vi "ReportPart.vi"(6 "试验项目":enum32{"静态标定", "动态优化", "程序复检", "程序固化"}(ring), 8 "error in":errorcluster, 9 "索引":i32=3, 10 "合格":T1, 11 "report in":refnum<class "NI_report.lvclass">) -> (0 "error out 2":errorcluster caption="error out", 1 "索引OUT":i32, 3 "report out":refnum<class "NI_report.lvclass">)   [LabVIEW 2020]
uses:
  <vilib>/Utility/NIReport.llb/NI_report.lvclass
  OK.ctl
  <vilib>/Utility/NIReport.llb/image depth.ctl
  <vilib>/addons/_office/_exclsub.llb/font.ctl
  Global_Variable/Global.vi
  <vilib>/Utility/NIReport.llb/Append Report Text (str wrap).vi
  <vilib>/addons/_office/word.llb/Word Easy Table (str).vi
  Global_Variable/A180648.vi
  <vilib>/Utility/NIReport.llb/NI_ReportGenerationCore.lvlib
  <vilib>/addons/_office/NI_ReportGenerationToolkit.lvlib
  <vilib>/Utility/NIReport.llb/Word/NI_Word.lvclass
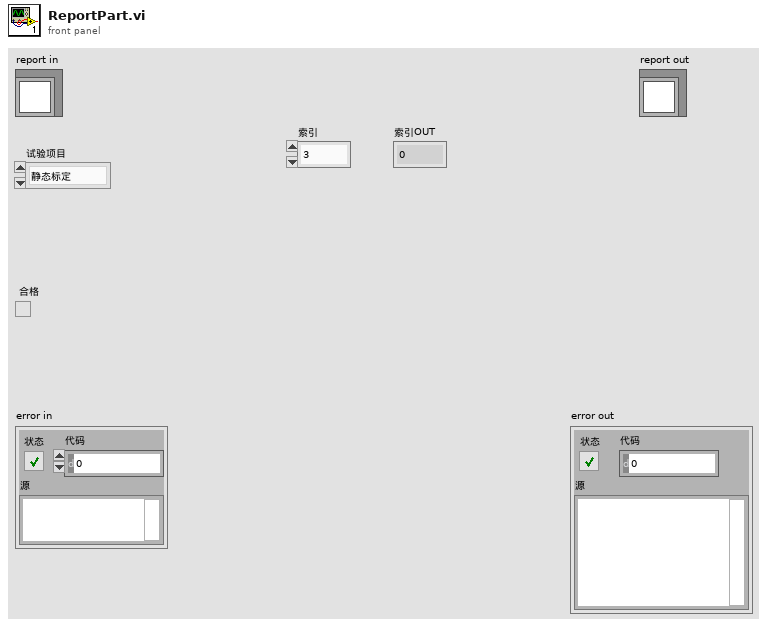
[diagram p1: front panel]
types:
  T1 = typedef "OK.ctl" = bool
  T2 = cluster{"Charset (-1)":i16, "Weight (-1)":i16, "Name":string, "Size":string}
  T3 = cluster{"Italic":enum16{"Italic Unchanged", "Italic On", "Italic Off"}, "Strike Through":enum16{"Strike Through Unchanged", "Strike Through On", "Strike Through Off"}, "Underline":enum16{"Underline Unchanged", "Underline On", "Underline Off"}, "Bold":enum16{"Bold Unchanged", "Bold On", "Bold Off"}}
  T4 = typedef "NI_ReportGenerationToolkit.lvlib/font.ctl" = cluster{"font name":string, "font size":dbl, "bold":u16, "italic":u16, "underline":u16, "strike through":u16, "font color":u32}
  T5 = typedef "NI_ReportGenerationCore.lvlib/image depth.ctl" = u16
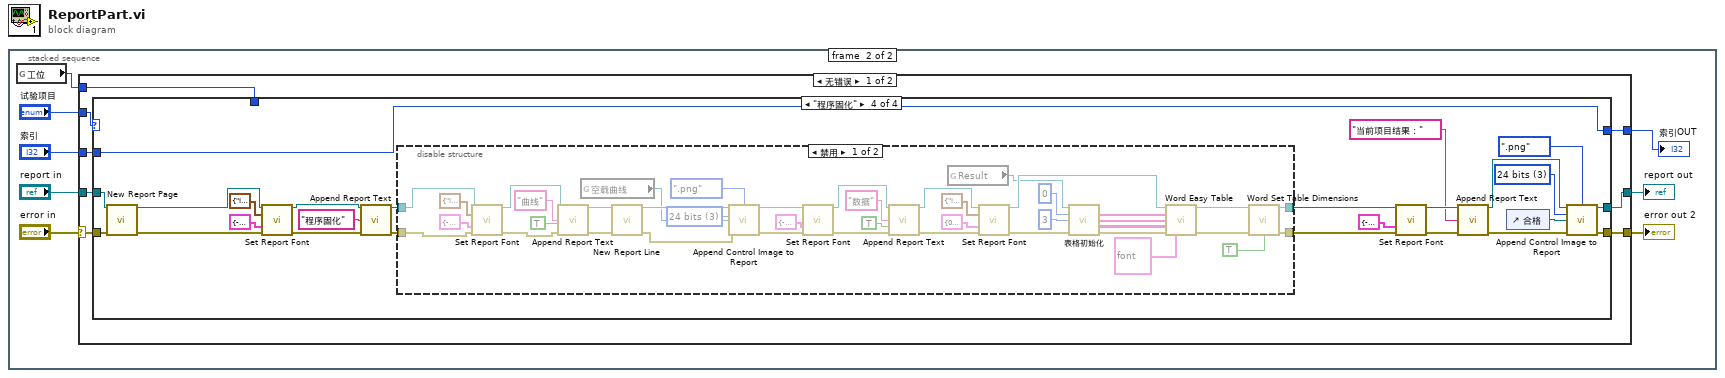
[diagram p0: block diagram]
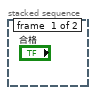
[diagram p2: hidden frame]
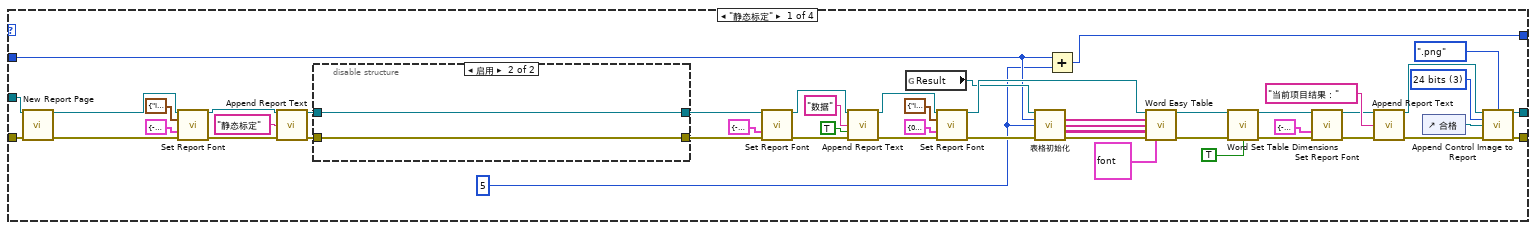
[diagram p3: hidden frame]
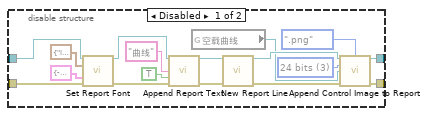
[diagram p4: hidden frame]
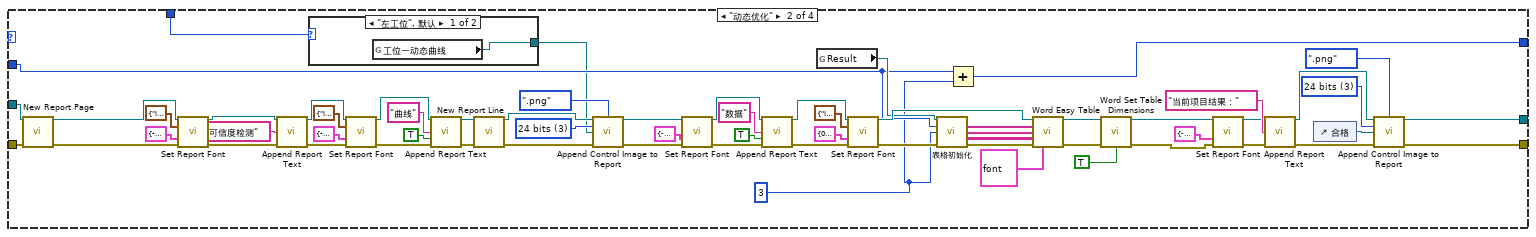
[diagram p5: hidden frame]
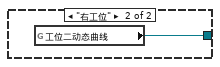
[diagram p6: hidden frame]
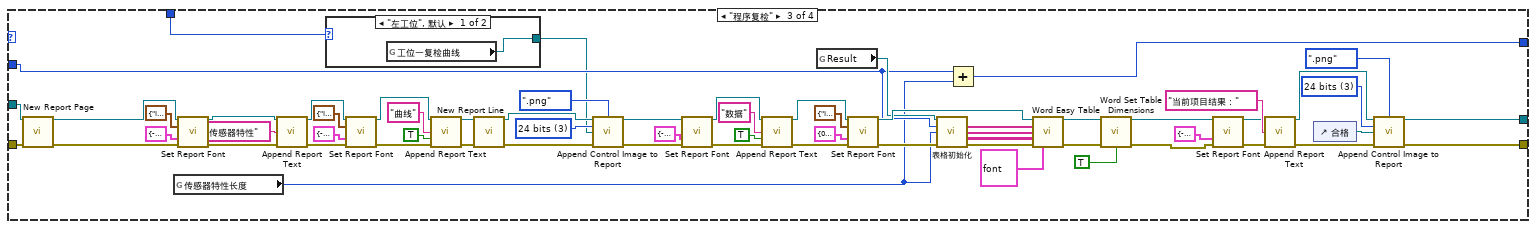
[diagram p7: hidden frame]
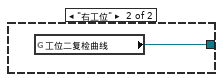
[diagram p8: hidden frame]
diagram:
  n1 = stacked-sequence {
    frame #0 {
    }
    frame #1 {
      n2 = global read "Global.vi" "工位"() -> (w1:enum16{"左工位", "右工位"})
      n3 = case shown="无错误" "error in" {
        selector: "error in" -> [w16 w285]
        tunnel: [w15 w285] -> w7
        tunnel: "试验项目" -> [w12 _]
        tunnel: [w14 w284] -> w5
        tunnel: "report in" -> [w13 w284]
        tunnel: "索引" -> [w11 w283]
        tunnel: [w10 w283] -> w2
        tunnel: w1 -> [w9 _]
        frame No Error {
          n4 = case shown="\"程序固化\"" w12 {
            tunnel: w16 -> [w59 w141 w206 w233]
            tunnel: [w54 w136 w201 w228] -> w15
            tunnel: [w23 w93 w158 w220] -> w14
            tunnel: w13 -> [w22 w92 w157 w219]
            tunnel: w11 -> [w19 w89 w154 w215]
            tunnel: [w18 w88 w153 w215] -> w10
            tunnel: w9 -> [_ w87 w152 _]
            frame "静态标定" {
              w17 = 5
              w52 = T5 3 items=["B&W", "4 bits", "8 bits", "24 bits"] ("image depth")
              n5 = call-dynamic "New Report Page.vi"("report in"=w22, "error in (no error)"=w59) -> ("report out"=w57:refnum<class "NI_report.lvclass">, "error out"=w58:errorcluster)  [unwired: 12 in]
              n6 = call-dynamic "Set Report Font.vi"("report in"=w57, "text options"=T3 {"Italic"=enum."Italic Unchanged", "Strike Through"=enum."Strike Through Unchanged", "Underline"=enum."Underline Unchanged", "Bold"=enum."Bold On"}, "font settings"=T2 {"Charset (-1)"=-1, "Weight (-1)"=-1, "Name"="楷体", "Size"="16 "}, "error in (no error)"=w58) -> ("report out"=w65:refnum<class "NI_report.lvclass">, "error out"=w64:errorcluster)  [unwired: 9 in, 1 out]
              n7 = call-poly <vilib>:"Append Report Text.vi"("report in"=w65, "text"="静态标定", "error in (no error)"=w64) -> ("report out"=w61:refnum<class "NI_report.lvclass">, "error out"=w60:errorcluster)  [unwired: 9 in, 2 out]
              n8 = disable-structure shown="启用" {
                disable-tunnel: w61 -> [w82 w84]
                disable-tunnel: w60 -> [w81 w83]
                disable-tunnel: [w77 w84] -> w41
                disable-tunnel: [w76 w83] -> w39
                frame Disabled {
                  w78 = T5 3 items=["B&W", "4 bits", "8 bits", "24 bits"] ("image depth")
                  n9 = call-dynamic "Set Report Font.vi"("report in"=w82, "text options"=T3 {"Italic"=enum."Italic Unchanged", "Strike Through"=enum."Strike Through Unchanged", "Underline"=enum."Underline Unchanged", "Bold"=enum."Bold Off"}, "font settings"=T2 {"Charset (-1)"=-1, "Weight (-1)"=-1, "Name"="宋体", "Size"="12 "}, "error in (no error)"=w81) -> ("report out"=w73:refnum<class "NI_report.lvclass">, "error out"=w70:errorcluster)  [unwired: 9 in, 1 out]
                  n10 = call-poly <vilib>:"Append Report Text.vi"("report in"=w73, "text"="曲线", "append on new line? (F)"=TRUE, "error in (no error)"=w70) -> ("report out"=w72:refnum<class "NI_report.lvclass">, "error out"=w71:errorcluster)  [unwired: 8 in, 2 out]
                  n11 = global read "A180648.vi" "空载曲线"() -> (w66:refnum<vi>)
                  n12 = call-dynamic "New Report Line.vi"("report in"=w72, "error in (no error)"=w71) -> ("report out"=w79:refnum<class "NI_report.lvclass">, "error out"=w80:errorcluster)  [unwired: 12 in]
                  n13 = call-dynamic "Append Control Image to Report.vi"("report in"=w79, "image file type (.jpg)"=enum16{".jpg", ".png"}.".png", "image depth"=w78, "ctrl reference"=w66, "error in (no error)"=w80) -> ("report out"=w77:refnum<class "NI_report.lvclass">, "error out"=w76:errorcluster)  [unwired: 7 in, 2 out]
                }
                frame Enabled {
                }
              }
              n14 = call-dynamic "Set Report Font.vi"("report in"=w41, "font settings"=T2 {"Charset (-1)"=-1, "Weight (-1)"=-1, "Name"="宋体", "Size"="12 "}, "error in (no error)"=w39) -> ("report out"=w42:refnum<class "NI_report.lvclass">, "error out"=w40:errorcluster)  [unwired: 10 in, 1 out]
              n15 = call-poly <vilib>:"Append Report Text.vi"("report in"=w42, "text"="数据", "append on new line? (F)"=TRUE, "error in (no error)"=w40) -> ("report out"=w26:refnum<class "NI_report.lvclass">, "error out"=w25:errorcluster)  [unwired: 8 in, 2 out]
              n16 = global read "Global.vi" "Result"() -> (w24:refnum<vi>)
              n17 = call-dynamic "Set Report Font.vi"("report in"=w26, "text options"=T3 {"Italic"=enum."Italic Unchanged", "Strike Through"=enum."Strike Through Unchanged", "Underline"=enum."Underline Unchanged", "Bold"=enum."Bold Unchanged"}, "font settings"=T2 {"Charset (-1)"=0, "Weight (-1)"=-1, "Name"="微软雅黑", "Size"="12 "}, "error in (no error)"=w25) -> ("report out"=w28:refnum<class "NI_report.lvclass">, "error out"=w27:errorcluster)  [unwired: 9 in, 1 out]
              n18 = call "表格初始化.vi"("表格引用"=w24, "索引"=w19, "长度"=w17, "错误输入（无错误）"=w27) -> ("行首字符串[]"=w30:string[], "列首字符串[]"=w29:string[], "文本数据"=w32:string[][], "错误输出"=w35:errorcluster)  [unwired: 7 in, 1 out]
              n19 = Add(x=w19, y=w17) -> (x+y=w18:i32)
              n20 = call-poly <vilib>:"Word Easy Table.vi"("report in"=w28, "row headers"=w30, "column headers"=w29, "data"=w32, "error in (no error)"=w35, "font"=T4 {"font name"="宋体", "font size"=12.0, "bold"=2, "italic"=2, "underline"=2, "strike through"=2, "font color"=16777216}) -> ("report out"=w33:refnum<class "NI_report.lvclass">, "error out"=w34:errorcluster)  [unwired: 7 in, 1 out]
              n21 = call <vilib>:"Word Set Table Dimensions.vi"("report in"=w33, "error in (no error)"=w34, "fit to page width? (F)"=TRUE) -> ("report out"=w47:refnum<class "NI_report.lvclass">, "error out"=w46:errorcluster)  [unwired: 11 in]
              n22 = call-dynamic "Set Report Font.vi"("report in"=w47, "font settings"=T2 {"Charset (-1)"=-1, "Weight (-1)"=-1, "Name"="宋体", "Size"="16 "}, "error in (no error)"=w46) -> ("report out"=w50:refnum<class "NI_report.lvclass">, "error out"=w51:errorcluster)  [unwired: 10 in, 1 out]
              n23 = call-poly <vilib>:"Append Report Text.vi"("report in"=w50, "text"="当前项目结果：", "error in (no error)"=w51) -> ("report out"=w56:refnum<class "NI_report.lvclass">, "error out"=w55:errorcluster)  [unwired: 9 in, 2 out]
              n24 = control-ref of="合格"() -> (w21:refnum<vi>)
              n25 = call-dynamic "Append Control Image to Report.vi"("report in"=w56, "image file type (.jpg)"=enum16{".jpg", ".png"}.".png", "image depth"=w52, "ctrl reference"=w21, "error in (no error)"=w55) -> ("report out"=w23:refnum<class "NI_report.lvclass">, "error out"=w54:errorcluster)  [unwired: 7 in, 2 out]
            }
            frame "动态优化" {
              w85 = 3
              w125 = T5 3 items=["B&W", "4 bits", "8 bits", "24 bits"] ("image depth")
              w134 = T5 3 items=["B&W", "4 bits", "8 bits", "24 bits"] ("image depth")
              n26 = call-dynamic "New Report Page.vi"("report in"=w92, "error in (no error)"=w141) -> ("report out"=w139:refnum<class "NI_report.lvclass">, "error out"=w140:errorcluster)  [unwired: 12 in]
              n27 = call-dynamic "Set Report Font.vi"("report in"=w139, "text options"=T3 {"Italic"=enum."Italic Unchanged", "Strike Through"=enum."Strike Through Unchanged", "Underline"=enum."Underline Unchanged", "Bold"=enum."Bold On"}, "font settings"=T2 {"Charset (-1)"=-1, "Weight (-1)"=-1, "Name"="楷体", "Size"="16 "}, "error in (no error)"=w140) -> ("report out"=w147:refnum<class "NI_report.lvclass">, "error out"=w146:errorcluster)  [unwired: 9 in, 1 out]
              n28 = call-poly <vilib>:"Append Report Text.vi"("report in"=w147, "text"="可信度检测", "error in (no error)"=w146) -> ("report out"=w143:refnum<class "NI_report.lvclass">, "error out"=w142:errorcluster)  [unwired: 9 in, 2 out]
              n29 = case shown="\"左工位\", 默认" w87 {
                tunnel: [w148 w149] -> w86
                frame "左工位", Default {
                  n30 = global read "A180648.vi" "工位一动态曲线"() -> (w148:refnum<vi>)
                }
                frame "右工位" {
                  n31 = global read "A180648.vi" "工位二动态曲线"() -> (w149:refnum<vi>)
                }
              }
              n32 = call-dynamic "Set Report Font.vi"("report in"=w143, "text options"=T3 {"Italic"=enum."Italic Unchanged", "Strike Through"=enum."Strike Through Unchanged", "Underline"=enum."Underline Unchanged", "Bold"=enum."Bold Off"}, "font settings"=T2 {"Charset (-1)"=-1, "Weight (-1)"=-1, "Name"="宋体", "Size"="12 "}, "error in (no error)"=w142) -> ("report out"=w112:refnum<class "NI_report.lvclass">, "error out"=w109:errorcluster)  [unwired: 9 in, 1 out]
              n33 = call-poly <vilib>:"Append Report Text.vi"("report in"=w112, "text"="曲线", "append on new line? (F)"=TRUE, "error in (no error)"=w109) -> ("report out"=w111:refnum<class "NI_report.lvclass">, "error out"=w110:errorcluster)  [unwired: 8 in, 2 out]
              n34 = call-dynamic "New Report Line.vi"("report in"=w111, "error in (no error)"=w110) -> ("report out"=w126:refnum<class "NI_report.lvclass">, "error out"=w127:errorcluster)  [unwired: 12 in]
              n35 = call-dynamic "Append Control Image to Report.vi"("report in"=w126, "image file type (.jpg)"=enum16{".jpg", ".png"}.".png", "image depth"=w125, "ctrl reference"=w86, "error in (no error)"=w127) -> ("report out"=w120:refnum<class "NI_report.lvclass">, "error out"=w118:errorcluster)  [unwired: 7 in, 2 out]
              n36 = call-dynamic "Set Report Font.vi"("report in"=w120, "font settings"=T2 {"Charset (-1)"=-1, "Weight (-1)"=-1, "Name"="宋体", "Size"="12 "}, "error in (no error)"=w118) -> ("report out"=w121:refnum<class "NI_report.lvclass">, "error out"=w119:errorcluster)  [unwired: 10 in, 1 out]
              n37 = call-poly <vilib>:"Append Report Text.vi"("report in"=w121, "text"="数据", "append on new line? (F)"=TRUE, "error in (no error)"=w119) -> ("report out"=w96:refnum<class "NI_report.lvclass">, "error out"=w95:errorcluster)  [unwired: 8 in, 2 out]
              n38 = global read "Global.vi" "Result"() -> (w94:refnum<vi>)
              n39 = call-dynamic "Set Report Font.vi"("report in"=w96, "text options"=T3 {"Italic"=enum."Italic Unchanged", "Strike Through"=enum."Strike Through Unchanged", "Underline"=enum."Underline Unchanged", "Bold"=enum."Bold Unchanged"}, "font settings"=T2 {"Charset (-1)"=0, "Weight (-1)"=-1, "Name"="微软雅黑", "Size"="12 "}, "error in (no error)"=w95) -> ("report out"=w98:refnum<class "NI_report.lvclass">, "error out"=w97:errorcluster)  [unwired: 9 in, 1 out]
              n40 = call "表格初始化.vi"("表格引用"=w94, "索引"=w89, "长度"=w85, "错误输入（无错误）"=w97) -> ("行首字符串[]"=w101:string[], "列首字符串[]"=w100:string[], "文本数据"=w103:string[][], "错误输出"=w106:errorcluster)  [unwired: 7 in, 1 out]
              n41 = Add(x=w89, y=w85) -> (x+y=w88:i32)
              n42 = call-poly <vilib>:"Word Easy Table.vi"("report in"=w98, "row headers"=w101, "column headers"=w100, "data"=w103, "error in (no error)"=w106, "font"=T4 {"font name"="宋体", "font size"=12.0, "bold"=2, "italic"=2, "underline"=2, "strike through"=2, "font color"=16777216}) -> ("report out"=w104:refnum<class "NI_report.lvclass">, "error out"=w105:errorcluster)  [unwired: 7 in, 1 out]
              n43 = call <vilib>:"Word Set Table Dimensions.vi"("report in"=w104, "error in (no error)"=w105, "fit to page width? (F)"=TRUE) -> ("report out"=w129:refnum<class "NI_report.lvclass">, "error out"=w128:errorcluster)  [unwired: 11 in]
              n44 = call-dynamic "Set Report Font.vi"("report in"=w129, "font settings"=T2 {"Charset (-1)"=-1, "Weight (-1)"=-1, "Name"="宋体", "Size"="16 "}, "error in (no error)"=w128) -> ("report out"=w132:refnum<class "NI_report.lvclass">, "error out"=w133:errorcluster)  [unwired: 10 in, 1 out]
              n45 = call-poly <vilib>:"Append Report Text.vi"("report in"=w132, "text"="当前项目结果：", "error in (no error)"=w133) -> ("report out"=w138:refnum<class "NI_report.lvclass">, "error out"=w137:errorcluster)  [unwired: 9 in, 2 out]
              n46 = control-ref of="合格"() -> (w91:refnum<vi>)
              n47 = call-dynamic "Append Control Image to Report.vi"("report in"=w138, "image file type (.jpg)"=enum16{".jpg", ".png"}.".png", "image depth"=w134, "ctrl reference"=w91, "error in (no error)"=w137) -> ("report out"=w93:refnum<class "NI_report.lvclass">, "error out"=w136:errorcluster)  [unwired: 7 in, 2 out]
            }
            frame "程序复检" {
              w190 = T5 3 items=["B&W", "4 bits", "8 bits", "24 bits"] ("image depth")
              w199 = T5 3 items=["B&W", "4 bits", "8 bits", "24 bits"] ("image depth")
              n48 = call-dynamic "New Report Page.vi"("report in"=w157, "error in (no error)"=w206) -> ("report out"=w204:refnum<class "NI_report.lvclass">, "error out"=w205:errorcluster)  [unwired: 12 in]
              n49 = global read "检测结果.vi" "传感器特性长度"() -> (w150:i32)
              n50 = call-dynamic "Set Report Font.vi"("report in"=w204, "text options"=T3 {"Italic"=enum."Italic Unchanged", "Strike Through"=enum."Strike Through Unchanged", "Underline"=enum."Underline Unchanged", "Bold"=enum."Bold On"}, "font settings"=T2 {"Charset (-1)"=-1, "Weight (-1)"=-1, "Name"="楷体", "Size"="16 "}, "error in (no error)"=w205) -> ("report out"=w212:refnum<class "NI_report.lvclass">, "error out"=w211:errorcluster)  [unwired: 9 in, 1 out]
              n51 = call-poly <vilib>:"Append Report Text.vi"("report in"=w212, "text"="传感器特性", "error in (no error)"=w211) -> ("report out"=w208:refnum<class "NI_report.lvclass">, "error out"=w207:errorcluster)  [unwired: 9 in, 2 out]
              n52 = case shown="\"左工位\", 默认" w152 {
                tunnel: [w213 w214] -> w151
                frame "左工位", Default {
                  n53 = global read "A180648.vi" "工位一复检曲线"() -> (w213:refnum<vi>)
                }
                frame "右工位" {
                  n54 = global read "A180648.vi" "工位二复检曲线"() -> (w214:refnum<vi>)
                }
              }
              n55 = call-dynamic "Set Report Font.vi"("report in"=w208, "text options"=T3 {"Italic"=enum."Italic Unchanged", "Strike Through"=enum."Strike Through Unchanged", "Underline"=enum."Underline Unchanged", "Bold"=enum."Bold Off"}, "font settings"=T2 {"Charset (-1)"=-1, "Weight (-1)"=-1, "Name"="宋体", "Size"="12 "}, "error in (no error)"=w207) -> ("report out"=w177:refnum<class "NI_report.lvclass">, "error out"=w174:errorcluster)  [unwired: 9 in, 1 out]
              n56 = call-poly <vilib>:"Append Report Text.vi"("report in"=w177, "text"="曲线", "append on new line? (F)"=TRUE, "error in (no error)"=w174) -> ("report out"=w176:refnum<class "NI_report.lvclass">, "error out"=w175:errorcluster)  [unwired: 8 in, 2 out]
              n57 = call-dynamic "New Report Line.vi"("report in"=w176, "error in (no error)"=w175) -> ("report out"=w191:refnum<class "NI_report.lvclass">, "error out"=w192:errorcluster)  [unwired: 12 in]
              n58 = call-dynamic "Append Control Image to Report.vi"("report in"=w191, "image file type (.jpg)"=enum16{".jpg", ".png"}.".png", "image depth"=w190, "ctrl reference"=w151, "error in (no error)"=w192) -> ("report out"=w185:refnum<class "NI_report.lvclass">, "error out"=w183:errorcluster)  [unwired: 7 in, 2 out]
              n59 = call-dynamic "Set Report Font.vi"("report in"=w185, "font settings"=T2 {"Charset (-1)"=-1, "Weight (-1)"=-1, "Name"="宋体", "Size"="12 "}, "error in (no error)"=w183) -> ("report out"=w186:refnum<class "NI_report.lvclass">, "error out"=w184:errorcluster)  [unwired: 10 in, 1 out]
              n60 = call-poly <vilib>:"Append Report Text.vi"("report in"=w186, "text"="数据", "append on new line? (F)"=TRUE, "error in (no error)"=w184) -> ("report out"=w161:refnum<class "NI_report.lvclass">, "error out"=w160:errorcluster)  [unwired: 8 in, 2 out]
              n61 = global read "Global.vi" "Result"() -> (w159:refnum<vi>)
              n62 = call-dynamic "Set Report Font.vi"("report in"=w161, "text options"=T3 {"Italic"=enum."Italic Unchanged", "Strike Through"=enum."Strike Through Unchanged", "Underline"=enum."Underline Unchanged", "Bold"=enum."Bold Unchanged"}, "font settings"=T2 {"Charset (-1)"=0, "Weight (-1)"=-1, "Name"="微软雅黑", "Size"="12 "}, "error in (no error)"=w160) -> ("report out"=w163:refnum<class "NI_report.lvclass">, "error out"=w162:errorcluster)  [unwired: 9 in, 1 out]
              n63 = call "表格初始化.vi"("表格引用"=w159, "索引"=w154, "长度"=w150, "错误输入（无错误）"=w162) -> ("行首字符串[]"=w166:string[], "列首字符串[]"=w165:string[], "文本数据"=w168:string[][], "错误输出"=w171:errorcluster)  [unwired: 7 in, 1 out]
              n64 = Add(x=w154, y=w150) -> (x+y=w153:i32)
              n65 = call-poly <vilib>:"Word Easy Table.vi"("report in"=w163, "row headers"=w166, "column headers"=w165, "data"=w168, "error in (no error)"=w171, "font"=T4 {"font name"="宋体", "font size"=12.0, "bold"=2, "italic"=2, "underline"=2, "strike through"=2, "font color"=16777216}) -> ("report out"=w169:refnum<class "NI_report.lvclass">, "error out"=w170:errorcluster)  [unwired: 7 in, 1 out]
              n66 = call <vilib>:"Word Set Table Dimensions.vi"("report in"=w169, "error in (no error)"=w170, "fit to page width? (F)"=TRUE) -> ("report out"=w194:refnum<class "NI_report.lvclass">, "error out"=w193:errorcluster)  [unwired: 11 in]
              n67 = call-dynamic "Set Report Font.vi"("report in"=w194, "font settings"=T2 {"Charset (-1)"=-1, "Weight (-1)"=-1, "Name"="宋体", "Size"="16 "}, "error in (no error)"=w193) -> ("report out"=w197:refnum<class "NI_report.lvclass">, "error out"=w198:errorcluster)  [unwired: 10 in, 1 out]
              n68 = call-poly <vilib>:"Append Report Text.vi"("report in"=w197, "text"="当前项目结果：", "error in (no error)"=w198) -> ("report out"=w203:refnum<class "NI_report.lvclass">, "error out"=w202:errorcluster)  [unwired: 9 in, 2 out]
              n69 = control-ref of="合格"() -> (w156:refnum<vi>)
              n70 = call-dynamic "Append Control Image to Report.vi"("report in"=w203, "image file type (.jpg)"=enum16{".jpg", ".png"}.".png", "image depth"=w199, "ctrl reference"=w156, "error in (no error)"=w202) -> ("report out"=w158:refnum<class "NI_report.lvclass">, "error out"=w201:errorcluster)  [unwired: 7 in, 2 out]
            }
            frame "程序固化" {
              w227 = T5 3 items=["B&W", "4 bits", "8 bits", "24 bits"] ("image depth")
              n71 = call-dynamic "New Report Page.vi"("report in"=w219, "error in (no error)"=w233) -> ("report out"=w231:refnum<class "NI_report.lvclass">, "error out"=w232:errorcluster)  [unwired: 12 in]
              n72 = call-dynamic "Set Report Font.vi"("report in"=w231, "text options"=T3 {"Italic"=enum."Italic Unchanged", "Strike Through"=enum."Strike Through Unchanged", "Underline"=enum."Underline Unchanged", "Bold"=enum."Bold On"}, "font settings"=T2 {"Charset (-1)"=-1, "Weight (-1)"=-1, "Name"="楷体", "Size"="16 "}, "error in (no error)"=w232) -> ("report out"=w239:refnum<class "NI_report.lvclass">, "error out"=w238:errorcluster)  [unwired: 9 in, 1 out]
              n73 = call-poly <vilib>:"Append Report Text.vi"("report in"=w239, "text"="程序固化", "error in (no error)"=w238) -> ("report out"=w235:refnum<class "NI_report.lvclass">, "error out"=w234:errorcluster)  [unwired: 9 in, 2 out]
              n74 = disable-structure shown="禁用" {
                disable-tunnel: w235 -> [w280 w282]
                disable-tunnel: w234 -> [w279 w281]
                disable-tunnel: [w278 w282] -> w222
                disable-tunnel: [w277 w281] -> w221
                frame Disabled {
                  w250 = T5 3 items=["B&W", "4 bits", "8 bits", "24 bits"] ("image depth")
                  n75 = call-dynamic "Set Report Font.vi"("report in"=w280, "text options"=T3 {"Italic"=enum."Italic Unchanged", "Strike Through"=enum."Strike Through Unchanged", "Underline"=enum."Underline Unchanged", "Bold"=enum."Bold Off"}, "font settings"=T2 {"Charset (-1)"=-1, "Weight (-1)"=-1, "Name"="宋体", "Size"="12 "}, "error in (no error)"=w279) -> ("report out"=w247:refnum<class "NI_report.lvclass">, "error out"=w244:errorcluster)  [unwired: 9 in, 1 out]
                  n76 = call-poly <vilib>:"Append Report Text.vi"("report in"=w247, "text"="曲线", "append on new line? (F)"=TRUE, "error in (no error)"=w244) -> ("report out"=w246:refnum<class "NI_report.lvclass">, "error out"=w245:errorcluster)  [unwired: 8 in, 2 out]
                  n77 = global read "A180648.vi" "空载曲线"() -> (w240:refnum<vi>)
                  n78 = call-dynamic "New Report Line.vi"("report in"=w246, "error in (no error)"=w245) -> ("report out"=w251:refnum<class "NI_report.lvclass">, "error out"=w252:errorcluster)  [unwired: 12 in]
                  n79 = call-dynamic "Append Control Image to Report.vi"("report in"=w251, "image file type (.jpg)"=enum16{".jpg", ".png"}.".png", "image depth"=w250, "ctrl reference"=w240, "error in (no error)"=w252) -> ("report out"=w272:refnum<class "NI_report.lvclass">, "error out"=w270:errorcluster)  [unwired: 7 in, 2 out]
                  n80 = call-dynamic "Set Report Font.vi"("report in"=w272, "font settings"=T2 {"Charset (-1)"=-1, "Weight (-1)"=-1, "Name"="宋体", "Size"="12 "}, "error in (no error)"=w270) -> ("report out"=w273:refnum<class "NI_report.lvclass">, "error out"=w271:errorcluster)  [unwired: 10 in, 1 out]
                  n81 = call-poly <vilib>:"Append Report Text.vi"("report in"=w273, "text"="数据", "append on new line? (F)"=TRUE, "error in (no error)"=w271) -> ("report out"=w257:refnum<class "NI_report.lvclass">, "error out"=w256:errorcluster)  [unwired: 8 in, 2 out]
                  n82 = global read "Global.vi" "Result"() -> (w255:refnum<vi>)
                  n83 = call-dynamic "Set Report Font.vi"("report in"=w257, "text options"=T3 {"Italic"=enum."Italic Unchanged", "Strike Through"=enum."Strike Through Unchanged", "Underline"=enum."Underline Unchanged", "Bold"=enum."Bold Unchanged"}, "font settings"=T2 {"Charset (-1)"=0, "Weight (-1)"=-1, "Name"="微软雅黑", "Size"="12 "}, "error in (no error)"=w256) -> ("report out"=w259:refnum<class "NI_report.lvclass">, "error out"=w258:errorcluster)  [unwired: 9 in, 1 out]
                  n84 = call "表格初始化.vi"("表格引用"=w255, "索引"=0, "长度"=3, "错误输入（无错误）"=w258) -> ("行首字符串[]"=w261:string[], "列首字符串[]"=w260:string[], "文本数据"=w263:string[][], "错误输出"=w266:errorcluster)  [unwired: 7 in, 1 out]
                  n85 = call-poly <vilib>:"Word Easy Table.vi"("report in"=w259, "row headers"=w261, "column headers"=w260, "data"=w263, "error in (no error)"=w266, "font"=T4 {"font name"="宋体", "font size"=12.0, "bold"=2, "italic"=2, "underline"=2, "strike through"=2, "font color"=16777216}) -> ("report out"=w264:refnum<class "NI_report.lvclass">, "error out"=w265:errorcluster)  [unwired: 7 in, 1 out]
                  n86 = call <vilib>:"Word Set Table Dimensions.vi"("report in"=w264, "error in (no error)"=w265, "fit to page width? (F)"=TRUE) -> ("report out"=w278:refnum<class "NI_report.lvclass">, "error out"=w277:errorcluster)  [unwired: 11 in]
                }
                frame Enabled {
                }
              }
              n87 = call-dynamic "Set Report Font.vi"("report in"=w222, "font settings"=T2 {"Charset (-1)"=-1, "Weight (-1)"=-1, "Name"="宋体", "Size"="16 "}, "error in (no error)"=w221) -> ("report out"=w225:refnum<class "NI_report.lvclass">, "error out"=w226:errorcluster)  [unwired: 10 in, 1 out]
              n88 = call-poly <vilib>:"Append Report Text.vi"("report in"=w225, "text"="当前项目结果：", "error in (no error)"=w226) -> ("report out"=w230:refnum<class "NI_report.lvclass">, "error out"=w229:errorcluster)  [unwired: 9 in, 2 out]
              n89 = control-ref of="合格"() -> (w218:refnum<vi>)
              n90 = call-dynamic "Append Control Image to Report.vi"("report in"=w230, "image file type (.jpg)"=enum16{".jpg", ".png"}.".png", "image depth"=w227, "ctrl reference"=w218, "error in (no error)"=w229) -> ("report out"=w220:refnum<class "NI_report.lvclass">, "error out"=w228:errorcluster)  [unwired: 7 in, 2 out]
            }
          }
        }
        frame Error {
        }
      }
      "error out 2" <- w7
      "report out" <- w5
      "索引OUT" <- w2
    }
  }
